vi "Disconnect CAN Adapter.vi"(8 "error in":errorcluster, 11 "CANopen Master in":refnum<class "CANopen Master.lvclass">) -> (0 "error out":errorcluster, 3 "CANopen Master out":refnum<class "CANopen Master.lvclass">)   [LabVIEW 2024, in "CANopen Master.lvlib" / "CANopen Master.lvclass"]
uses:
  CANopen Master.lvclass
  CANopen Master.lvclass/CANopen Master.ctl
  HAL/Source/Interfaces/IClose/IClose.lvclass
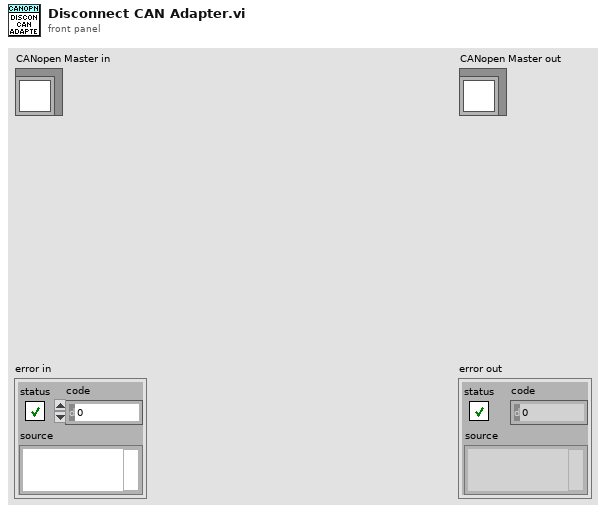
[diagram p1: front panel]
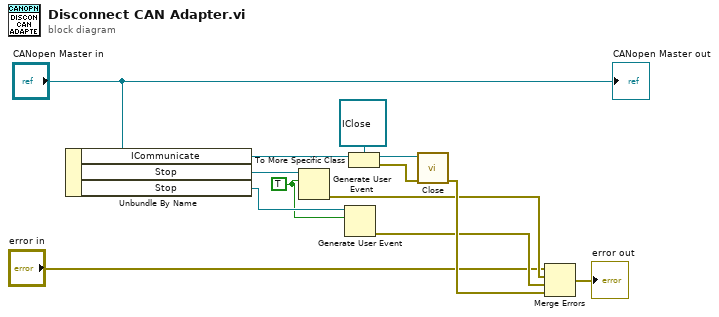
[diagram p0: block diagram]
diagram:
  w4 = TRUE ("event data")
  n1 = Unbundle By Name("CANopen Master in") -> ("ICommunicate"=w11:refnum<class "ICommunicate.lvclass">, "Stop"=w12:refnum<user-event>, "Stop"=w5:refnum<user-event>)
  n2 = Generate User Event(user event=w12, event data cluster=w4) -> (error out=w3:errorcluster)  [unwired: 2 in, 1 out]
  n3 = Generate User Event(user event=w5, event data cluster=w4) -> (error out=w2:errorcluster)  [unwired: 2 in, 1 out]
  n4 = To More Specific Class(target class=refnum<class "IClose.lvclass"> refnum ("IClose.lvclass"), reference=w11) -> (specific class reference=w10:refnum<class "IClose.lvclass">, error out=w9:errorcluster)  [unwired: 1 in]
  n5 = call-dynamic "Close.vi"("error in"=w9, "IClose in"=w10) -> ("error out"=w8:errorcluster)  [unwired: 8 in, 1 out]
  n6 = Merge Errors("error in", w3, w2, w8) -> (→"error out":errorcluster)
  "CANopen Master out" <- "CANopen Master in"
